vi "Assignment1_2.vi"() -> ()   [LabVIEW 2025]
panel:
  out "C":i32
  in  "Stop":bool
  in  "Operations":T1(ring)
  in  "N":i32
  in  "M":i32
  # "Do Some Opearation Based on \"Select Operation\""
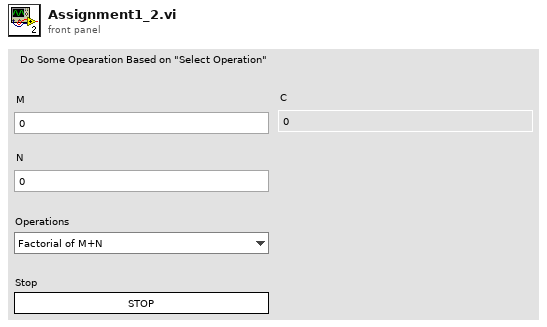
[diagram p1: front panel]
types:
  T1 = enum16{"Factorial of M+N ", "Sum of factorials of first M natural number", "Sum of factorials of first N whole numbers ", "Greater of M and N "}
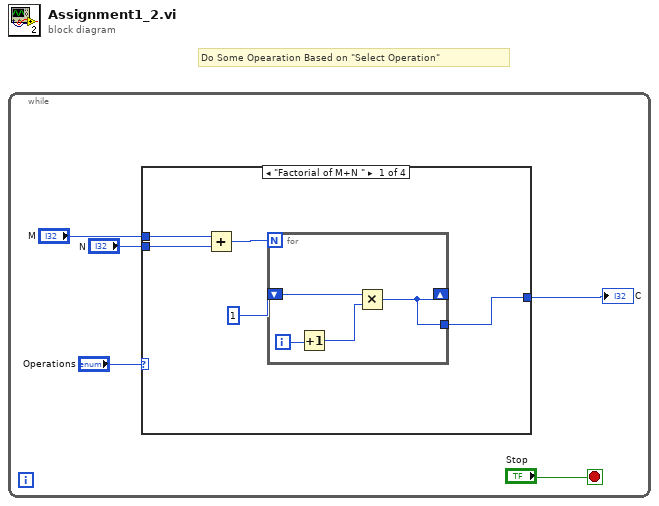
[diagram p0: block diagram]
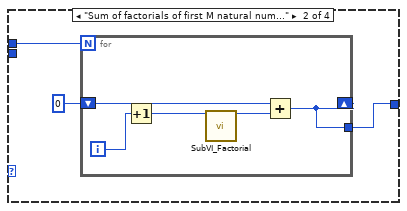
[diagram p2: hidden frame]
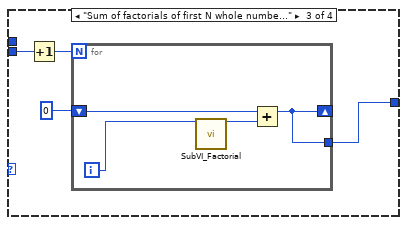
[diagram p3: hidden frame]
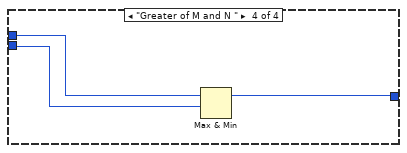
[diagram p4: hidden frame]
diagram:
  # "Do Some Opearation Based on \"Select Operation\""
  n1 = while {
    stop <- "Stop" stop-if-true
    n2 = case shown="\"Factorial of M+N \"" "Operations" {
      tunnel: "M" -> [w10 w17 _ w33]
      tunnel: "N" -> [w7 _ w24 w32]
      tunnel: [w6 w15 w23 w31] -> w1
      frame "Factorial of M+N " {
        n3 = Add(x=w10, y=w7) -> (x+y=w9:i32)
        n4 = for {
          N: w9 -> [_]
          shift-right: [w11] -> _
          shift-left: 1 -> [w12]
          tunnel: [w11] -> w6
          i -> [w14]
          n5 = Increment(x=w14) -> (x+1=w13:i32)
          n6 = Multiply(x=w12, y=w13) -> (x*y=w11:i32)
        }
      }
      frame "Sum of factorials of first M natural number" {
        n7 = for {
          N: w17 -> [_]
          shift-right: [w18] -> _
          shift-left: 0 -> [w19]
          tunnel: [w18] -> w15
          i -> [w22]
          n8 = Increment(x=w22) -> (x+1=w21:i32)
          n9 = call "SubVI_Factorial.vi"("Input"=w21) -> ("Factorial"=w20:i32)  [unwired: 14 in]
          n10 = Add(x=w19, y=w20) -> (x+y=w18:i32)
        }
      }
      frame "Sum of factorials of first N whole numbers " {
        n11 = Increment(x=w24) -> (x+1=w25:i32)
        n12 = for {
          N: w25 -> [_]
          shift-right: [w27] -> _
          shift-left: 0 -> [w29]
          tunnel: [w27] -> w23
          i -> [w28]
          n13 = call "SubVI_Factorial.vi"("Input"=w28) -> ("Factorial"=w30:i32)  [unwired: 14 in]
          n14 = Add(x=w29, y=w30) -> (x+y=w27:i32)
        }
      }
      frame "Greater of M and N " {
        n15 = Max & Min(x=w33, y=w32) -> (max(x,y)=w31:i32)  [unwired: 1 out]
      }
    }
    "C" <- w1
  }
